vi "Close Loader Handle.vi"(8 "error in (no error)":errorcluster, 11 "Loaders":T1[](array[typedef])) -> (0 "error out":errorcluster)   [LabVIEW 2021, in "CIFPluginManager.lvclass"]
uses:
  CIFPluginManager.lvclass
  typedef/Loaders.ctl
  typedef/Loader Type.ctl
  <vilib>/gRPC/LabVIEW gRPC Library/Shared/grpcId.ctl
  CIFUtilities/CIFLogs/Typedef/Message Type.ctl
  CIFCore/Common/Typedef/Errors.ctl
  <vilib>/CIF Foundation/CIF Utilities/Errors/Append Error Location.vi
  CIFPluginManager.lvclass/CIFPluginManager.ctl
  CIFCore/Common/CIFCoreCommon.lvlib
  CIFUtilities/CIFLogs/CIFLogs.lvlib
  CIFPluginLoader/gRPC/CIF_Plugin_Loader_Client_Wrapper/CIFPluginLoaderClientWrapper.lvlib
  <vilib>/gRPC/LabVIEW gRPC Library/grpc-lvsupport-release.lvlib
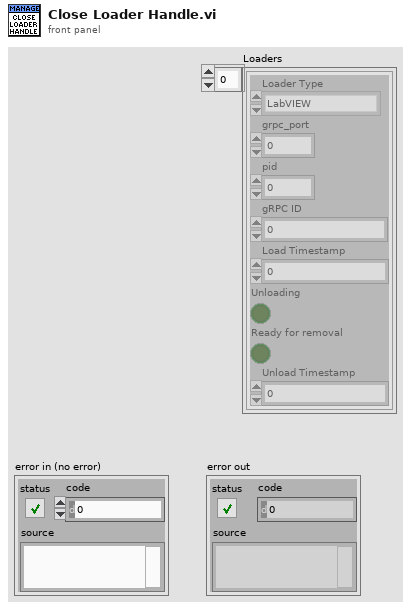
[diagram p1: front panel]
types:
  T1 = typedef "CIFPluginManager.lvclass/Loaders.ctl" = cluster{"Loader Type":T2, "grpc_port":i32, "pid":u32, "gRPC ID":T3, "Load Timestamp":i64, "Unloading":bool, "Ready for removal":bool, "Unload Timestamp":i64}
  T2 = typedef "CIFPluginManager.lvclass/Loader Type.ctl" = enum16{"LabVIEW"}
  T3 = typedef "grpc-lvsupport-release.lvlib/grpcId.ctl" = u64
  T4 = typedef "CIFLogs.lvlib/Message Type.ctl" = enum16{"Error", "Information", "Print Terminal", "Configuration"}
  T5 = typedef "CIFCoreCommon.lvlib/Errors.ctl" = enum16{"Invalid Clock ID", "Long Sleep", "gRPC Server Not Found", "Config Parse", "Timestamp Wrap", "Delayed Execution", "Duplicate Channel", "Missing Channel", "Incorrect Type", "Flatten Error", "Unflatten Data", "Unique Name", "Plugin Not Found", "Plugin Type Not Found", "Plugin Version Not Found", "Manager Not Found", "Numerical Issue", "Time Jump", "Clock ID Match", "Channel Length", "Plugin Connection", "gRPC Server Connection", "PPL Name Match", "Build", "Config Log Parse", "Plugin Load", "UI Subpanel Load", "Python Name", "Invalid Name", "Unable to Change Ch Buffer", "Failed Kill"}
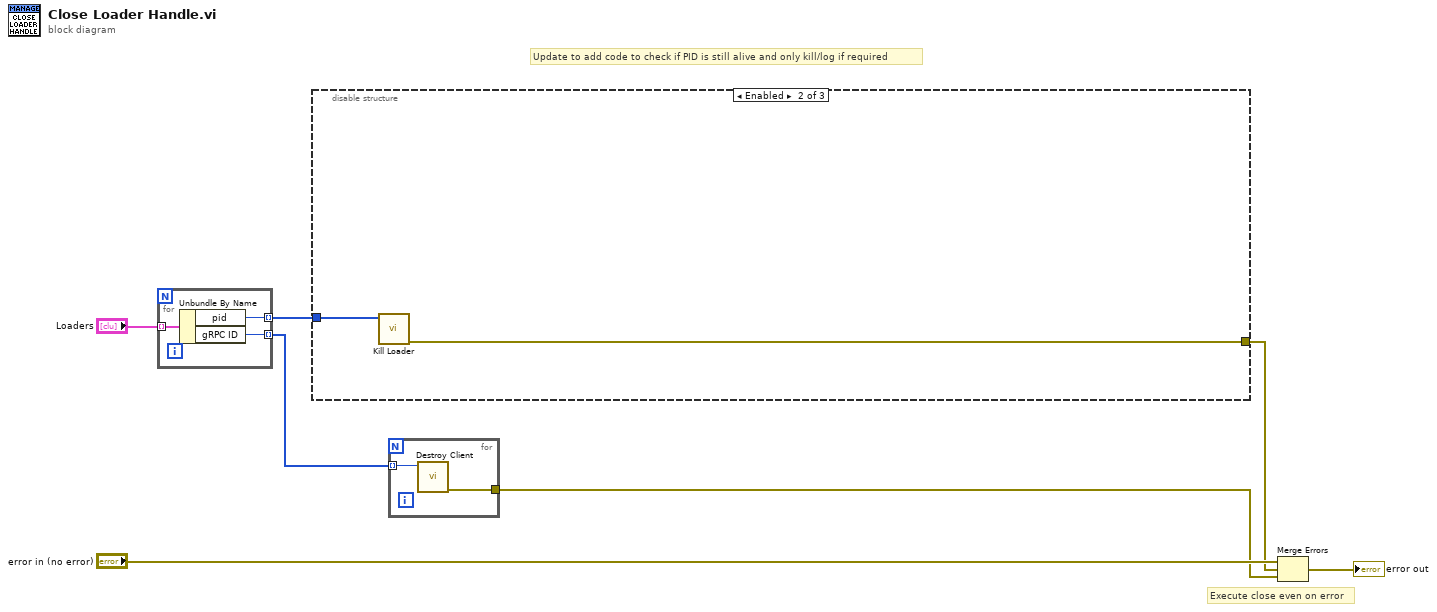
[diagram p0: block diagram]
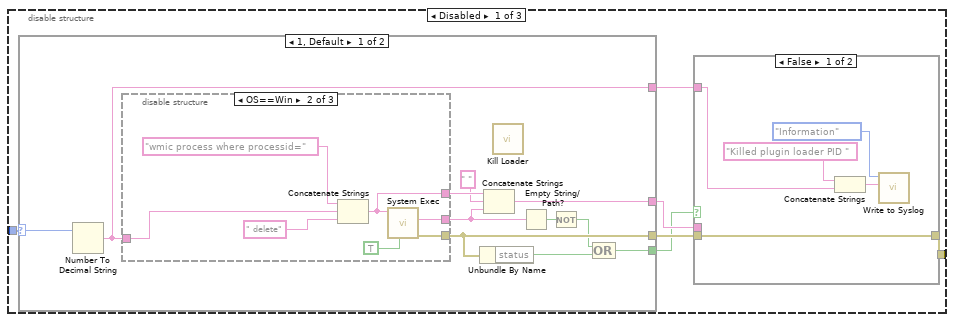
[diagram p2: hidden frame]
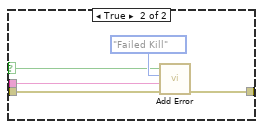
[diagram p3: hidden frame]
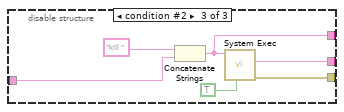
[diagram p5: hidden frame]
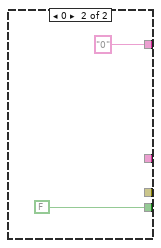
[diagram p6: hidden frame]
diagram:
  # "Update to add code to check if PID is still alive and only kill/log if required"
  # "Execute close even on error"
  n1 = for {
    tunnel: [w10] -> w4 mode=indexing
    tunnel: [w9] -> w2 mode=indexing
    tunnel: "Loaders" -> [w8] mode=indexing
    n2 = Unbundle By Name(w8) -> ("pid"=w9:u32, "gRPC ID"=w10:T3)
  }
  n3 = disable-structure shown="Enabled" {
    disable-tunnel: [w15 w54 _] -> w3
    disable-tunnel: w2 -> [w13 w53 _]
    frame Disabled {
      n4 = case shown="1, Default" w13 {
        selector: w13 -> [w32 _]
        tunnel: [w31 _] -> w16
        tunnel: [w35 _] -> w14
        tunnel: [w28 FALSE] -> w12
        tunnel: [w27 "0"] -> w11
        frame 1, Default {
          n5 = Number To Decimal String(number=w32) -> (decimal integer string=w27:string)  [unwired: 1 in]
          n6 = disable-structure shown="OS==Win" {
            disable-tunnel: w27 -> [_ w44 w49]
            disable-tunnel: [_ w42 w47] -> w31
            disable-tunnel: [_ w41 w46] -> w34
            disable-tunnel: [_ w40 w45] -> w37
            frame condition #0 {
            }
            frame condition #1 (active) {
              n7 = Concatenate Strings("wmic process where processid=", w44, " delete") -> (w40:string)
              n8 = call <vilib>:"System Exec.vi"("run minimized? (F)"=TRUE, "command line"=w40) -> ("error out"=w42:errorcluster, "standard error"=w41:string)  [unwired: 6 in, 2 out]
            }
            frame condition #2 {
              n9 = Concatenate Strings("kill ", w49) -> (w45:string)
              n10 = call <vilib>:"System Exec.vi"("run minimized? (F)"=TRUE, "command line"=w45) -> ("error out"=w47:errorcluster, "standard error"=w46:string)  [unwired: 6 in, 2 out]
            }
          }
          n11 = Unbundle By Name(w31) -> ("status"=w30:bool)
          n12 = Concatenate Strings(w37, " ", w34) -> (w35:string)
          n13 = call "Kill Loader.vi"() -> ()  [unwired: 9 in, 3 out]
          n14 = Empty String/Path?(string/path=w34) -> (empty?=w33:bool)
          n15 = Not(x=w33) -> (.not. x?=w29:bool)
          n16 = Compound Arithmetic op=OR(w29, w30) -> (w28:bool)
        }
        frame 0 {
        }
      }
      n17 = case shown="False" w12 {
        selector: w12 -> [_ w22]
        tunnel: w16 -> [w20 w26]
        tunnel: [w20 w25] -> w15
        tunnel: w14 -> [_ w24]
        tunnel: w11 -> [w17 _]
        frame False {
          n18 = Concatenate Strings("Killed plugin loader PID " ("message"), w17) -> (w18:string)
          n19 = call "Write to Syslog.vi"("message"=w18, "CIF Message Type"=Message_Type."Information") -> ()  [unwired: 9 in, 1 out]
        }
        frame True {
          n20 = call "Add Error.vi"("error in (no error)"=w26, "String to Append"=w24, "Error"=Errors."Failed Kill", "Insert Error"=w22) -> ("error out"=w25:errorcluster)  [unwired: 7 in]
        }
      }
    }
    frame Enabled {
      n21 = call "Kill Loader.vi"("PIDs"=w53) -> ("error out"=w54:errorcluster)  [unwired: 8 in, 2 out]
    }
    frame Disabled {
    }
  }
  n22 = for {
    tunnel: [w56] -> w5
    tunnel: w4 -> [w55] mode=indexing
    n23 = call "Destroy Client.vi"("gRPC ID"=w55) -> ("error out"=w56:errorcluster)  [unwired: 10 in]
  }
  n24 = Merge Errors("error in (no error)", w3, w5) -> (→"error out":errorcluster)
